vi "XML_AppendSubContent.vi"(10 "Append Content":T1, 11 "XML in":T1) -> (3 "XML out":T1)   [LabVIEW 2017]
doc: "Appends Append Content before the closing tag of the outermost element in XML in, so a child element can be added to an existing document."
uses:
  _XML--String.ctl
  _openG/_reuse_openG.lvlib
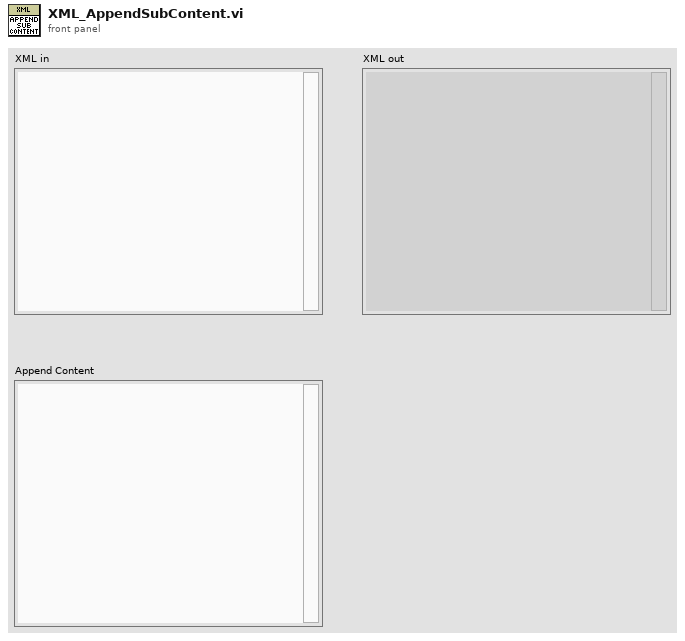
[diagram p1: front panel]
types:
  T1 = typedef "_XML--String.ctl" = string
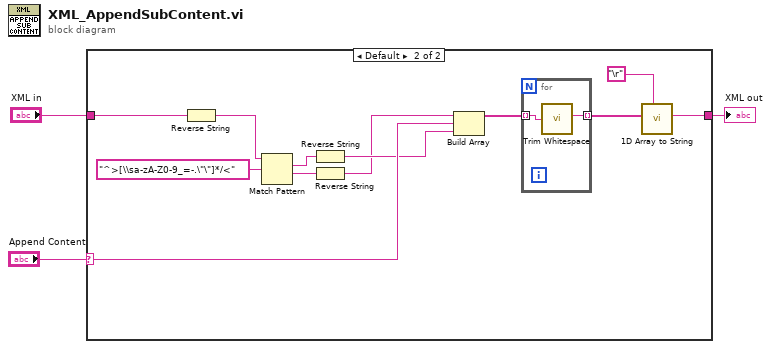
[diagram p0: block diagram]
diagram:
  n1 = case shown="Default" "Append Content" {
    selector: "Append Content" -> [_ w11]
    tunnel: [w4 w14] -> w3
    tunnel: "XML in" -> [w4 w13]
    frame "" {
    }
    frame Default {
      n2 = Reverse String(1:w13) -> (0:w8:T1)
      n3 = Match Pattern(string=w8, regular expression="^>[\\sa-zA-Z0-9_=-.\"\"]*/<" ("string")) -> (match substring=w5:T1, after substring=w12:T1)  [unwired: 1 in, 2 out]
      n4 = Reverse String(1:w5) -> (0:w10:T1)
      n5 = Reverse String(1:w12) -> (0:w9:T1)
      n6 = Build Array(w9, w11, w10) -> (w6:T1[])
      n7 = for {
        tunnel: [w18] -> w16 mode=indexing
        tunnel: w6 -> [w17] mode=indexing
        n8 = call <vilib>:"Trim Whitespace.vi"("string"=w17) -> ("trimmed string"=w18:string)  [unwired: 1 in]
      }
      n9 = call "1D Array to String.vi"("delimiter (Tab)"="\r", "Array of Strings"=w16) -> ("delimited string"=w14:string)  [unwired: 9 in]
    }
  }
  "XML out" <- w3
